vi "DAQmx.vi"() -> ()   [LabVIEW 2019]
uses:
  <vilib>/DAQmx/read.llb/DAQmx Read (Analog 1D Wfm NChan NSamp).vi
  <vilib>/DAQmx/create/channels.llb/DAQmx Create Channel (AI-Voltage-Basic).vi
  <vilib>/DAQmx/configure/timing.llb/DAQmx Timing (Sample Clock).vi
  <vilib>/DAQmx/miscellaneous.llb/DAQmx Fill In Error Info.vi
  <resource>/objmgr/ni.dex.rc
panel:
  out "error out":errorcluster
  out "Connected":bool
  out "Waveform Chart":waveform(dbl)[](graph)
  in  "stopbutton":bool
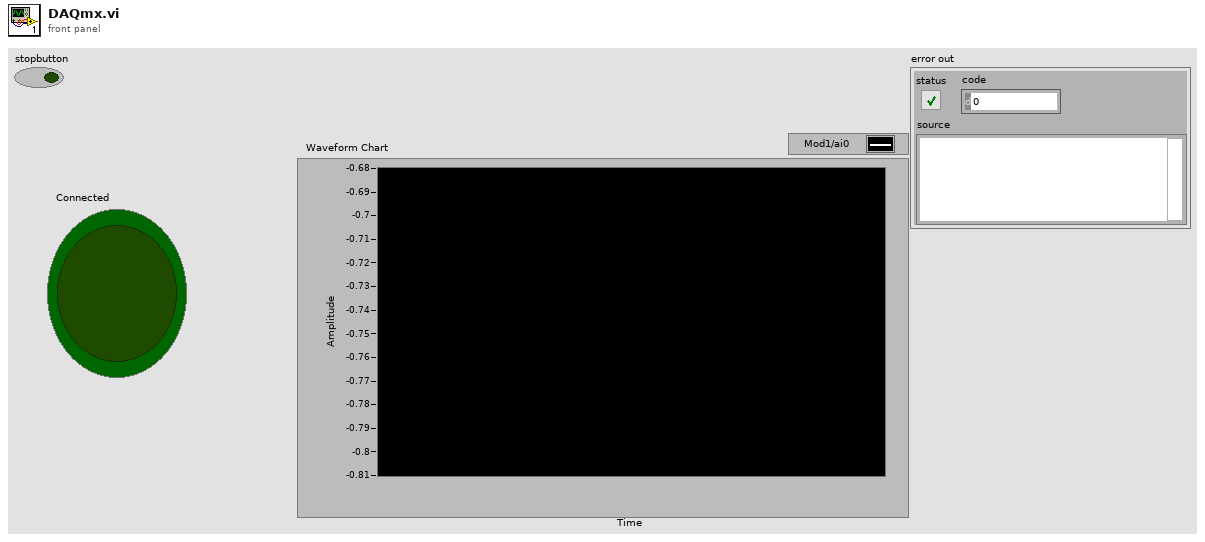
[diagram p1: front panel]
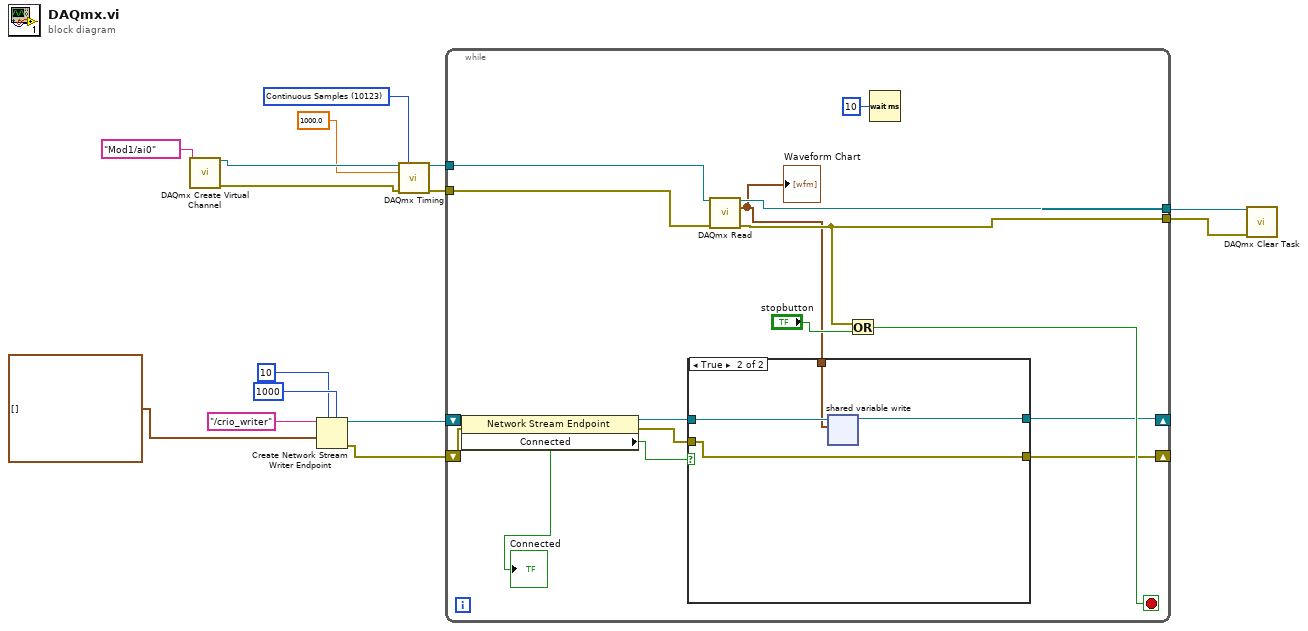
[diagram p0: block diagram]
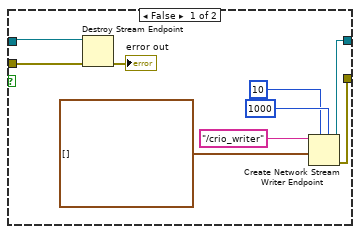
[diagram p2: hidden frame]
diagram:
  w11 = 10123 items=["Finite Samples"=10178, "Continuous Samples"=10123, "Hardware Timed Single Point"=12522] ("sample mode")
  n1 = call-poly <vilib>:"DAQmx Create Virtual Channel.vi"("physical channels"=tag "Mod1/ai0") -> ("task out"=w13:refnum<k21>, "error out"=w14:errorcluster)  [unwired: 13 in]
  n2 = Create Network Stream Writer Endpoint(5:1000 ("timeout in ms (-1)"), 7:10 ("writer buffer size"), 9:waveform(dbl)[] [] ("data"), 11:"/crio_writer" ("writer name")) -> (0:w2:errorcluster, 3:w5:refnum<k21>)  [unwired: 3 in]
  n3 = call-poly <vilib>:"DAQmx Timing.vi"("task/channels in"=w13, "sample mode"=w11, "rate"=1000.0, "error in"=w14) -> ("task out"=w10:refnum<k21>, "error out"=w9:errorcluster)  [unwired: 10 in]
  n4 = while {
    tunnel: w10 -> [w30]
    tunnel: w9 -> [w29]
    tunnel: [w25] -> w8
    tunnel: [w24] -> w7
    shift-right: [w21] -> _
    shift-left: w5 -> [w23]
    shift-right: [w16] -> _
    shift-left: w2 -> [w17]
    stop <- w28 stop-if-true
    n5 = property class="Network Stream Endpoint"(reference=w23, error in=w17) -> (reference out=w22:refnum<k21>, error out=w18:errorcluster, "Connected"=w19:bool)
    "Connected" <- w19
    n6 = call-poly <vilib>:"DAQmx Read.vi"("task/channels in"=w30, "error in"=w29) -> ("task out"=w25:refnum<k21>, "data"=w20:waveform(dbl)[], "error out"=w24:errorcluster)  [unwired: 11 in]
    "Waveform Chart" <- w20
    n7 = case shown="True" w19 {
      tunnel: w22 -> [w39 w43]
      tunnel: [w33 w42] -> w21
      tunnel: w20 -> [_ w40]
      tunnel: w18 -> [w38 w41]
      tunnel: [w32 w41] -> w16
      frame False {
        n8 = Destroy Stream Endpoint(8:w38, 11:w39) -> (0:→"error out":errorcluster)
        n9 = Create Network Stream Writer Endpoint(5:1000 ("timeout in ms (-1)"), 7:10 ("writer buffer size"), 9:waveform(dbl)[] [] ("data"), 11:"/crio_writer" ("writer name")) -> (0:w32:errorcluster, 3:w33:refnum<k21>)  [unwired: 3 in]
      }
      frame True {
        n10 = shared-variable-write(w43, w40) -> (w42:refnum<k21>)  [unwired: 2 in, 2 out]
      }
    }
    n11 = Or(x=w24, y="stopbutton") -> (x .or. y?=w28:bool)
    n12 = Wait (ms)(milliseconds to wait=u32 10) -> ()  [unwired: 1 out]
  }
  n13 = call <vilib>:"DAQmx Clear Task.vi"("task in"=w8, "error in"=w7) -> ()  [unwired: 13 in, 1 out]
